vi "HC MFR sw 3.vi"(8 "Increment":dbl, 9 "HC Conc %":dbl, 10 "C_HC":dbl, 11 "Flow rate":dbl) -> (3 "CO MFR":dbl)   [LabVIEW 2014]
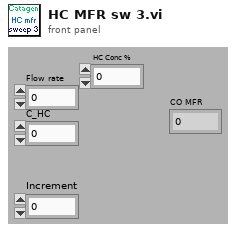
[diagram p1: front panel]
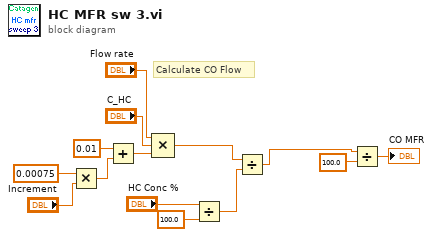
[diagram p0: block diagram]
diagram:
  # "Calculate CO Flow"
  n1 = Multiply(x=0.00075, y="Increment") -> (x*y=w8:dbl)
  n2 = Add(x=0.01, y=w8) -> (x+y=w7:dbl)
  n3 = Compound Arithmetic op=MULTIPLY("Flow rate", "C_HC", w7) -> (w5:dbl)
  n4 = Divide(x="HC Conc %", y=100.0) -> (x/y=w3:dbl)
  n5 = Divide(x=w5, y=w3) -> (x/y=w4:dbl)
  n6 = Divide(x=w4, y=100.0) -> (x/y=→"CO MFR":dbl)
